vi "Coherent command pre-processing L1.vi"(9 "Data":T2, 10 "Commands & Queries":T4, 11 "Coherent laser commands L1":T3(ring)) -> (2 "Data Type":T1, 3 "Command/Query string":string, 5 "Command validated ?":bool)   [LabVIEW 2020]
uses:
  Type defs/Commands List.ctl
  Type defs/data type.ctl
  Type defs/coherent commands list.ctl
  Type defs/coherent commands.ctl
  Type defs/Command mode.ctl
  Type defs/Command syntax.ctl
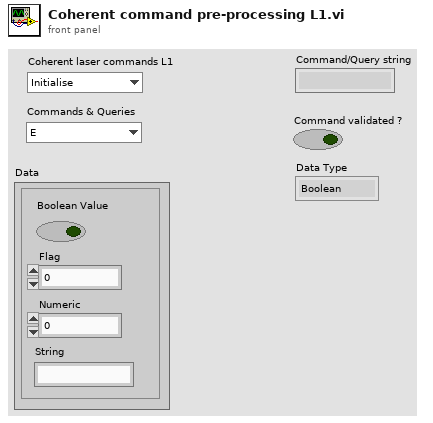
[diagram p1: front panel]
types:
  T1 = typedef "data type.ctl" = enum16{"Boolean", "Flag", "Numeric", "String", "Array"}
  T2 = cluster{"Boolean Value":bool, "Flag":i32, "Numeric":dbl, "String":string}
  T3 = enum16{"Initialise", "Get Command", "Set Command", "Close"}
  T4 = typedef "Commands List.ctl" = enum16{"E", "B", "FL", "HM", "L", "LBOH", "LBOOPT", "LFP", "PROMPT", "SM", "S", "VW", "VWS", "HB", "HBR", "REQ", "ALIGN", "K", "F", "FH", "UF", "PHLDC", "PZTMC", "PZTXC", "PZTYC", "PHLDP", "PZTMP", "PZTXP", "PZTYP", "PTRK", "MDLK", "PP", "TS", "STPRPOS", "C", "D1C", "D2C", "BT", "D1T", "D2T", "VT", "LBOT", "ET", "D1ST", "D2ST", "VST", "LBOST", "EST", "D1TD", "D2TD", "VD", "LBOD", "ED", "D1HST", "D2HST", "LRS", "D1SS", "D2SS", "VSS", "LBOSS", "ESS", "D1H", "D2H", "HH", "D1V", "D2V", "SV", "MB", "PI", "BV", "AMDLK", "PZTS", "TMAX", "TMIN", "ALIGNP", "ALIGNW", "PZTXCM", "PZTXCP", "PZTXPM", "PZTXPP", "PZTYCM", "PZTYCP", "PZTYPM", "PZTYPP", "RH", "SN", "ST", "GDDCURVE", "GDD", "GDDCURVEN", "SETCURVEN", "SETCURVEPT", "SAVECURVE", "DELCURVE", "CURVEN", "CURVEPT", "CURVE", "COMP", "HMCOMP", "GDDMAX", "GDDMIN"}
  T5 = typedef "coherent commands list.ctl" = T6[]
  T6 = typedef "coherent commands.ctl" = cluster{"Description":string, "Commands & Queries":T4, "Command Type":T7, "Data Type":T1, "Command Syntax":T8}
  T7 = typedef "Command mode.ctl" = enum16{"Read Only", "Write Only", "Read & Write"}
  T8 = typedef "Command syntax.ctl" = enum16{"Default", "Special"}
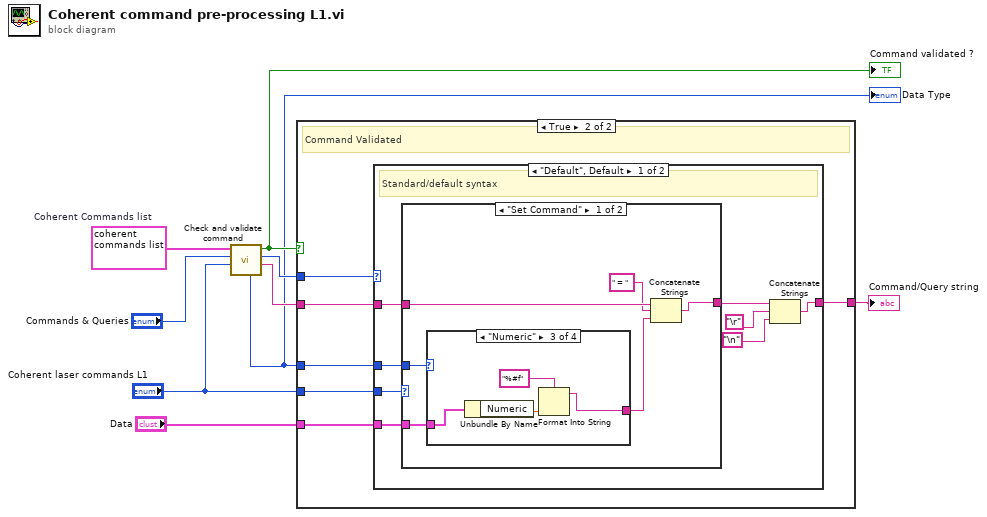
[diagram p0: block diagram]
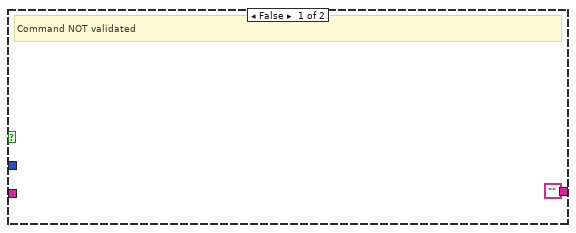
[diagram p2: hidden frame]
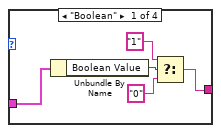
[diagram p3: hidden frame]
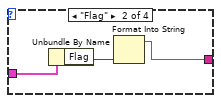
[diagram p4: hidden frame]
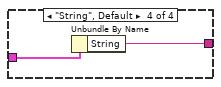
[diagram p5: hidden frame]
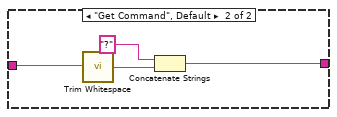
[diagram p6: hidden frame]
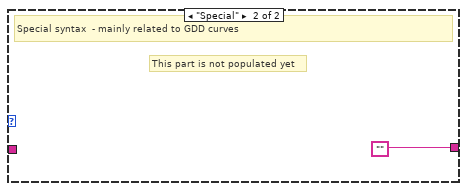
[diagram p7: hidden frame]
diagram:
  w8 = T5 [{"Description"="Changes echo settings", "Commands & Queries"=enum."E", "Command Type"=enum."Write Only", "Data Type"=enum."Boolean", "Command Syntax"=enum."Default"}, {"Description"="sets baudrate", "Commands & Queries"=enum."B", "Command Type"=enum."Write Only", "Data Type"=enum."Numeric", "Command Syntax"=enum."Default"}, {"Description"="Flash Verdi laser output below lasing threshold to allow single-frequency mode\nto recenter.\n", "Commands & Queries"=enum."FL", "Command Type"=enum."Write Only", "Data Type"=enum."Boolean", "Command Syntax"=enum."Default"}, {"Description"="Homes the tuning motor (this action can take between 3 to 30 seconds) OR provides the tuning motor status in read mode", "Commands & Queries"=enum."HM", "Command Type"=enum."Read & Write", "Data Type"=enum."Boolean", "Command Syntax"=enum."Default"}, {"Description"="changes laser mode from standby to ON or vice versa (with keyswitch in ON position). In read mode provides the Laser status\n", "Commands & Queries"=enum."L", "Command Type"=enum."Read & Write", "Data Type"=enum."Flag", "Command Syntax"=enum."Default"}, {"Description"="Turns LBO heater on/off. or indicates", "Commands & Queries"=enum."LBOH", "Command Type"=enum."Read & Write", "Data Type"=enum."Boolean", "Command Syntax"=enum."Default"}, {"Description"="Begins optimization routine.", "Commands & Queries"=enum."LBOOPT", "Command Type"=enum."Write Only", "Data Type"=enum."Boolean", "Command Syntax"=enum."Default"}, {"Description"="Turns \"CHAMELEON>\" prompt on/off.", "Commands & Queries"=enum."PROMPT", "Command Type"=enum."Write Only", "Data Type"=enum."Boolean", "Command Syntax"=enum."Default"}, {"Description"="Enables/disables search for modelocking. or displays status.", "Commands & Queries"=enum."SM", "Command Type"=enum."Read & Write", "Data Type"=enum."Boolean", "Command Syntax"=enum."Default"}, {"Description"="Changes state of the external shutter or shows the state of the shutter", "Commands & Queries"=enum."S", "Command Type"=enum."Read & Write", "Data Type"=enum."Boolean", "Command Syntax"=enum."Default"}, {"Description"="Set or display target wavelength in nanometers (nm)", "Commands & Queries"=enum."VW", "Command Type"=enum."Read & Write", "Data Type"=enum."Numeric", "Command Syntax"=enum."Default"}, {"Description"="Changes the Chameleon Ultra wavelength by the specified amount in nanometers (nm).\n", "Commands & Queries"=enum."VWS", "Command Type"=enum."Read & Write", "Data Type"=enum."Boolean", "Command Syntax"=enum."Default"}, {"Description"="When enabled, shuts the laser down if no RS-232 activity occurs within a time\nspecified by the heartbeat rate (HBR). n = 1 Enables heartbeat\n", "Commands & Queries"=enum."HB", "Command Type"=enum."Read & Write", "Data Type"=enum."Boolean", "Command Syntax"=enum."Default"}, {"Description"="Specifies to time-out period (between 1 to 100 seconds) for laser shut down in\nthe absence of RS-232 activity.", "Commands & Queries"=enum."HBR", "Command Type"=enum."Read & Write", "Data Type"=enum."Numeric", "Command Syntax"=enum."Default"}, {"Description"="Initiates recovery sequence.\nThis action can take up to 2 minutes to complete.", "Commands & Queries"=enum."REQ", "Command Type"=enum."Write Only", "Data Type"=enum."Boolean", "Command Syntax"=enum."Default"}, {"Description"="Accesses alignment mode\nn = 1 Enters alignment mode\nn = 0 Exits alignment mode", "Commands & Queries"=enum."ALIGN", "Command Type"=enum."Read & Write", "Data Type"=enum."Boolean", "Command Syntax"=enum."Default"}, {"Description"="Returns status of the keyswitch.", "Commands & Queries"=enum."K", "Command Type"=enum."Read Only", "Data Type"=enum."Boolean", "Command Syntax"=enum."Default"}, {"Description"="Returns a list of number codes of all active faults, separated by an \"&\" or\nReturns \"System OK\" if there are no active faults. Refer manual to look at the faults list\n", "Commands & Queries"=enum."F", "Command Type"=enum."Read Only", "Data Type"=enum."String", "Command Syntax"=enum."Default"}, {"Description"="Returns a list of number codes (see ?F) of all faults that have occurred since the\nlast laser on command, separated by an \"&\", or returns \"System OK\" if there are\nno latched faults. The \"laser on\" command or the EXIT button on the power\nsupply when the fault screen is active clears the fault history and fault screen.", "Commands & Queries"=enum."FH", "Command Type"=enum."Read Only", "Data Type"=enum."String", "Command Syntax"=enum."Default"}, {"Description"="Returns actual UF (Chameleon) power, nnn.nn, in milliwatts.", "Commands & Queries"=enum."UF", "Command Type"=enum."Read Only", "Data Type"=enum."Numeric", "Command Syntax"=enum."Default"}, {"Description"="Returns the status of the cavity peak hold: \n0 = Off\n1 = On\n", "Commands & Queries"=enum."PHLDC", "Command Type"=enum."Read Only", "Data Type"=enum."Boolean", "Command Syntax"=enum."Default"}, {"Description"="Returns the mode of the cavity PZT.\n0 = Auto\n1 = Manual\n", "Commands & Queries"=enum."PZTMC", "Command Type"=enum."Read Only", "Data Type"=enum."Boolean", "Command Syntax"=enum."Default"}, {"Description"="Returns the cavity PZT X (Rd) voltage, n.nn, in volts.", "Commands & Queries"=enum."PZTXC", "Command Type"=enum."Read Only", "Data Type"=enum."Numeric", "Command Syntax"=enum."Default"}, {"Description"="Returns the cavity PZT Y (Rd) voltage, n.nn, in volts.", "Commands & Queries"=enum."PZTYC", "Command Type"=enum."Read Only", "Data Type"=enum."Numeric", "Command Syntax"=enum."Default"}, {"Description"="Returns the status of the pump peak hold: \n0 = Off\n1 = On\n", "Commands & Queries"=enum."PHLDP", "Command Type"=enum."Read Only", "Data Type"=enum."Boolean", "Command Syntax"=enum."Default"}, {"Description"="Returns the mode of the pump PZT: \n0 = Auto\n1 = Manual\n", "Commands & Queries"=enum."PZTMP", "Command Type"=enum."Read Only", "Data Type"=enum."Boolean", "Command Syntax"=enum."Default"}, {"Description"="Returns pump PZT X (Rd) voltage, n.nn, in volts.", "Commands & Queries"=enum."PZTXP", "Command Type"=enum."Read Only", "Data Type"=enum."Numeric", "Command Syntax"=enum."Default"}, {"Description"="Returns pump PZT Y (Rd) voltage, n.nn, in volts.", "Commands & Queries"=enum."PZTYP", "Command Type"=enum."Read Only", "Data Type"=enum."Numeric", "Command Syntax"=enum."Default"}, {"Description"="Returns state of the PowerTrack : \n0 = Off\n1 = On", "Commands & Queries"=enum."PTRK", "Command Type"=enum."Read Only", "Data Type"=enum."Boolean", "Command Syntax"=enum."Default"}, {"Description"="Returns state of the Chameleon Ultra: \n0 = Off (Standby)\n1 = Modelocked\n2 = CW\n", "Commands & Queries"=enum."MDLK", "Command Type"=enum."Read Only", "Data Type"=enum."Flag", "Command Syntax"=enum."Default"}, {"Description"="Returns pump power setpoint as fraction of QS to CW pump band.", "Commands & Queries"=enum."PP", "Command Type"=enum."Read Only", "Data Type"=enum."Numeric", "Command Syntax"=enum."Default"}, {"Description"="Returns the tuning status:\n0 = Ready (i.e. no tuning operation being performed)\n1 = Tuning in progress\n2 = Search for Modelock in progress\n3 = Recovery operation in progress", "Commands & Queries"=enum."TS", "Command Type"=enum."Read Only", "Data Type"=enum."Flag", "Command Syntax"=enum."Default"}, {"Description"="Returns the position (counts) that the motor was last moved to for a desired\ntuning.\n", "Commands & Queries"=enum."STPRPOS", "Command Type"=enum."Read Only", "Data Type"=enum."Numeric", "Command Syntax"=enum."Default"}, {"Description"="Measured average diode current", "Commands & Queries"=enum."C", "Command Type"=enum."Read Only", "Data Type"=enum."Numeric", "Command Syntax"=enum."Default"}, {"Description"="Laser diode #1 measured current (A)", "Commands & Queries"=enum."D1C", "Command Type"=enum."Read Only", "Data Type"=enum."Numeric", "Command Syntax"=enum."Default"}, {"Description"="Laser diode #2 measured current (A)", "Commands & Queries"=enum."D2C", "Command Type"=enum."Read Only", "Data Type"=enum."Numeric", "Command Syntax"=enum."Default"}, {"Description"="Base plate temperature (deg C)", "Commands & Queries"=enum."BT", "Command Type"=enum."Read Only", "Data Type"=enum."Numeric", "Command Syntax"=enum."Default"}, {"Description"="Laser diode #1 measured temperature (deg C)", "Commands & Queries"=enum."D1T", "Command Type"=enum."Read Only", "Data Type"=enum."Numeric", "Command Syntax"=enum."Default"}, {"Description"="Laser diode #2 measured temperature (deg C)", "Commands & Queries"=enum."D2T", "Command Type"=enum."Read Only", "Data Type"=enum."Boolean", "Command Syntax"=enum."Default"}, {"Description"="Vanadate measured temperature (deg C)", "Commands & Queries"=enum."VT", "Command Type"=enum."Read Only", "Data Type"=enum."Numeric", "Command Syntax"=enum."Default"}, {"Description"="LBO temperature (deg C)", "Commands & Queries"=enum."LBOT", "Command Type"=enum."Read Only", "Data Type"=enum."Numeric", "Command Syntax"=enum."Default"}, {"Description"="Etalon measured temperature (deg C)", "Commands & Queries"=enum."ET", "Command Type"=enum."Read Only", "Data Type"=enum."Numeric", "Command Syntax"=enum."Default"}, {"Description"="Laser diode #1 set temperature (deg C)", "Commands & Queries"=enum."D1ST", "Command Type"=enum."Read Only", "Data Type"=enum."Numeric", "Command Syntax"=enum."Default"}, {"Description"="Laser diode #1 set temperature (deg C)", "Commands & Queries"=enum."D2ST", "Command Type"=enum."Read Only", "Data Type"=enum."Numeric", "Command Syntax"=enum."Default"}, {"Description"="Vanadate set temperature (deg C)", "Commands & Queries"=enum."VST", "Command Type"=enum."Read Only", "Data Type"=enum."Numeric", "Command Syntax"=enum."Default"}, {"Description"="LBO set temperature (deg C)", "Commands & Queries"=enum."LBOST", "Command Type"=enum."Read Only", "Data Type"=enum."Numeric", "Command Syntax"=enum."Default"}, {"Description"="Etalon set temperature (deg C)", "Commands & Queries"=enum."EST", "Command Type"=enum."Read Only", "Data Type"=enum."Numeric", "Command Syntax"=enum."Default"}, {"Description"="Laser diode #1 temperature servo drive setting", "Commands & Queries"=enum."D1TD", "Command Type"=enum."Read Only", "Data Type"=enum."Numeric", "Command Syntax"=enum."Default"}, {"Description"="Laser diode #2 temperature servo drive setting", "Commands & Queries"=enum."D2TD", "Command Type"=enum."Read Only", "Data Type"=enum."Numeric", "Command Syntax"=enum."Default"}, {"Description"="Vanadate temperature servo drive setting", "Commands & Queries"=enum."VD", "Command Type"=enum."Read Only", "Data Type"=enum."Numeric", "Command Syntax"=enum."Default"}, {"Description"="LBO temperature servo drive setting", "Commands & Queries"=enum."LBOD", "Command Type"=enum."Read Only", "Data Type"=enum."Numeric", "Command Syntax"=enum."Default"}, {"Description"="Etalon temperature servo drive setting", "Commands & Queries"=enum."ED", "Command Type"=enum."Read Only", "Data Type"=enum."Numeric", "Command Syntax"=enum."Default"}, {"Description"="Laser diode #1 heat sink measured temperature (deg C)", "Commands & Queries"=enum."D1HST", "Command Type"=enum."Read Only", "Data Type"=enum."Numeric", "Command Syntax"=enum."Default"}, {"Description"="Laser diode #2 heat sink measured temperature (deg C)", "Commands & Queries"=enum."D2HST", "Command Type"=enum."Read Only", "Data Type"=enum."Numeric", "Command Syntax"=enum."Default"}, {"Description"="Light loop servo status", "Commands & Queries"=enum."LRS", "Command Type"=enum."Read Only", "Data Type"=enum."Flag", "Command Syntax"=enum."Default"}, {"Description"="Diode #1 temperature servo status.", "Commands & Queries"=enum."D1SS", "Command Type"=enum."Read Only", "Data Type"=enum."Flag", "Command Syntax"=enum."Default"}, {"Description"="Diode #2 temperature servo status.", "Commands & Queries"=enum."D2SS", "Command Type"=enum."Read Only", "Data Type"=enum."Flag", "Command Syntax"=enum."Default"}, {"Description"="Vanadate temperature servo status", "Commands & Queries"=enum."VSS", "Command Type"=enum."Read Only", "Data Type"=enum."Flag", "Command Syntax"=enum."Default"}, {"Description"="LBO temperature servo status", "Commands & Queries"=enum."LBOSS", "Command Type"=enum."Read Only", "Data Type"=enum."Flag", "Command Syntax"=enum."Default"}, {"Description"="Etalon temperature servo status", "Commands & Queries"=enum."ESS", "Command Type"=enum."Read Only", "Data Type"=enum."Flag", "Command Syntax"=enum."Default"}, {"Description"="Operating hours of laser diode #1", "Commands & Queries"=enum."D1H", "Command Type"=enum."Read Only", "Data Type"=enum."Numeric", "Command Syntax"=enum."Default"}, {"Description"="Operating hours of laser diode #2", "Commands & Queries"=enum."D2H", "Command Type"=enum."Read Only", "Data Type"=enum."Numeric", "Command Syntax"=enum."Default"}, {"Description"="Power supply software", "Commands & Queries"=enum."SV", "Command Type"=enum."Read Only", "Data Type"=enum."Numeric", "Command Syntax"=enum."Default"}, {"Description"="Modem baud rate", "Commands & Queries"=enum."MB", "Command Type"=enum."Read Only", "Data Type"=enum."Numeric", "Command Syntax"=enum."Default"}, {"Description"="1 bar or 2 bar power supply", "Commands & Queries"=enum."PI", "Command Type"=enum."Read Only", "Data Type"=enum."Boolean", "Command Syntax"=enum."Default"}, {"Description"="Measured voltage across the battery.", "Commands & Queries"=enum."BV", "Command Type"=enum."Read Only", "Data Type"=enum."Numeric", "Command Syntax"=enum."Default"}, {"Description"="Auto mode lock routing", "Commands & Queries"=enum."AMDLK", "Command Type"=enum."Read Only", "Data Type"=enum."Boolean", "Command Syntax"=enum."Default"}, {"Description"="PTZ control state", "Commands & Queries"=enum."PZTS", "Command Type"=enum."Read Only", "Data Type"=enum."String", "Command Syntax"=enum."Default"}, {"Description"="Maximum available wavelength (nm)", "Commands & Queries"=enum."TMAX", "Command Type"=enum."Read Only", "Data Type"=enum."Numeric", "Command Syntax"=enum."Default"}, {"Description"="Minimum available wavelength (nm)", "Commands & Queries"=enum."TMIN", "Command Type"=enum."Read Only", "Data Type"=enum."Boolean", "Command Syntax"=enum."Default"}, {"Description"="Laser power available with alignment mode enabled (mW)", "Commands & Queries"=enum."ALIGNP", "Command Type"=enum."Read Only", "Data Type"=enum."Numeric", "Command Syntax"=enum."Default"}, {"Description"="Alignment mode laser wavelength", "Commands & Queries"=enum."ALIGNW", "Command Type"=enum."Read Only", "Data Type"=enum."Numeric", "Command Syntax"=enum."Default"}, {"Description"="Enable/disable input from front panel.", "Commands & Queries"=enum."LFP", "Command Type"=enum."Read & Write", "Data Type"=enum."Boolean", "Command Syntax"=enum."Default"}, {"Description"="X PZT position power map (% of available range)", "Commands & Queries"=enum."PZTXCM", "Command Type"=enum."Read Only", "Data Type"=enum."Numeric", "Command Syntax"=enum."Default"}, {"Description"="current cavity X PZT position (% of available range).", "Commands & Queries"=enum."PZTXCP", "Command Type"=enum."Read Only", "Data Type"=enum."Numeric", "Command Syntax"=enum."Default"}, {"Description"="X PZT position pump last power map", "Commands & Queries"=enum."PZTXPM", "Command Type"=enum."Read & Write", "Data Type"=enum."Numeric", "Command Syntax"=enum."Default"}, {"Description"="Current pump X PZT position (% of available range)", "Commands & Queries"=enum."PZTXPP", "Command Type"=enum."Read Only", "Data Type"=enum."Boolean", "Command Syntax"=enum."Default"}, {"Description"="Y PZT position power map (% of available range)", "Commands & Queries"=enum."PZTYCM", "Command Type"=enum."Read Only", "Data Type"=enum."Numeric", "Command Syntax"=enum."Default"}, {"Description"="current cavity Y PZT position (% of available range).", "Commands & Queries"=enum."PZTYCP", "Command Type"=enum."Read Only", "Data Type"=enum."Numeric", "Command Syntax"=enum."Default"}, {"Description"="Y PZT position pump last power map", "Commands & Queries"=enum."PZTYPM", "Command Type"=enum."Read Only", "Data Type"=enum."Numeric", "Command Syntax"=enum."Default"}, {"Description"="Current pump Y PZT position (% of available range)", "Commands & Queries"=enum."PZTYPP", "Command Type"=enum."Read Only", "Data Type"=enum."Boolean", "Command Syntax"=enum."Default"}, {"Description"="Relative humidity (%)", "Commands & Queries"=enum."RH", "Command Type"=enum."Read & Write", "Data Type"=enum."Numeric", "Command Syntax"=enum."Default"}, {"Description"="Chameleon serial number", "Commands & Queries"=enum."SN", "Command Type"=enum."Read Only", "Data Type"=enum."String", "Command Syntax"=enum."Default"}, {"Description"="Current status", "Commands & Queries"=enum."ST", "Command Type"=enum."Read Only", "Data Type"=enum."String", "Command Syntax"=enum."Default"}, {"Description"="GDD calibration curve number", "Commands & Queries"=enum."GDDCURVE", "Command Type"=enum."Read & Write", "Data Type"=enum."Numeric", "Command Syntax"=enum."Default"}, {"Description"="GDD value (fs2)", "Commands & Queries"=enum."GDD", "Command Type"=enum."Read & Write", "Data Type"=enum."Numeric", "Command Syntax"=enum."Default"}, {"Description"="GDD curve name", "Commands & Queries"=enum."GDDCURVEN", "Command Type"=enum."Read & Write", "Data Type"=enum."String", "Command Syntax"=enum."Default"}, {"Description"="Sets GDD curve name", "Commands & Queries"=enum."SETCURVEN", "Command Type"=enum."Read Only", "Data Type"=enum."String", "Command Syntax"=enum."Special"}, {"Description"="Curve ww point position (read manual)", "Commands & Queries"=enum."SETCURVEPT", "Command Type"=enum."Read Only", "Data Type"=enum."Numeric", "Command Syntax"=enum."Default"}, {"Description"="Save curve", "Commands & Queries"=enum."SAVECURVE", "Command Type"=enum."Write Only", "Data Type"=enum."Numeric", "Command Syntax"=enum."Default"}, {"Description"="delete curve", "Commands & Queries"=enum."DELCURVE", "Command Type"=enum."Write Only", "Data Type"=enum."Numeric", "Command Syntax"=enum."Default"}, {"Description"="Current curve name", "Commands & Queries"=enum."CURVEN", "Command Type"=enum."Read Only", "Data Type"=enum."String", "Command Syntax"=enum."Default"}, {"Description"="Curve ww point ", "Commands & Queries"=enum."CURVEPT", "Command Type"=enum."Read Only", "Data Type"=enum."Array", "Command Syntax"=enum."Special"}, {"Description"="Calibration points", "Commands & Queries"=enum."CURVE", "Command Type"=enum."Read Only", "Data Type"=enum."Array", "Command Syntax"=enum."Special"}, {"Description"="Pre compenstor enabled ?", "Commands & Queries"=enum."COMP", "Command Type"=enum."Read Only", "Data Type"=enum."Boolean", "Command Syntax"=enum."Default"}, {"Description"="Pre-compensator stepper ", "Commands & Queries"=enum."HMCOMP", "Command Type"=enum."Read Only", "Data Type"=enum."Boolean", "Command Syntax"=enum."Default"}, {"Description"="Max GDD value (at current wavelength or specified wavelength)", "Commands & Queries"=enum."GDDMAX", "Command Type"=enum."Read Only", "Data Type"=enum."Numeric", "Command Syntax"=enum."Special"}, {"Description"="Min GDD value (at current wavelength or specified wavelength)", "Commands & Queries"=enum."GDDMIN", "Command Type"=enum."Read Only", "Data Type"=enum."Numeric", "Command Syntax"=enum."Special"}]  # Coherent Commands list
  n1 = call "Check and validate command.vi"("Coherent laser commands L1"="Coherent laser commands L1", "Commands & Queries"="Commands & Queries", "Coherent Commands list"=w8) -> ("Command String"=w5:string, "Command Syntax"=w6:T8, "Command validated ?"=w7:bool, "Data Type"=w3:T1)  [unwired: 5 in]
  "Command validated ?" <- w7
  "Data Type" <- w3
  n2 = case shown="True" w7 {
    tunnel: w6 -> [_ w16]
    tunnel: w5 -> [_ w15]
    tunnel: "Coherent laser commands L1" -> [_ w14]
    tunnel: ["" w13] -> w2
    tunnel: "Data" -> [_ w12]
    tunnel: w3 -> [_ w11]
    frame False {
      # "Command NOT validated"
    }
    frame True {
      # "Command Validated"
      n3 = case shown="\"Default\", Default" w16 {
        tunnel: w15 -> [w23 _]
        tunnel: w14 -> [w24 _]
        tunnel: [w17 ""] -> w13
        tunnel: w12 -> [w22 _]
        tunnel: w11 -> [w21 _]
        frame "Default", Default {
          # "Standard/default syntax"
          n4 = case shown="\"Set Command\"" w24 {
            tunnel: w23 -> [w28 w48]
            tunnel: [w27 w45] -> w18
            tunnel: w22 -> [w29 _]
            tunnel: w21 -> [w30 _]
            frame "Set Command" {
              n5 = case shown="\"Numeric\"" w30 {
                tunnel: w29 -> [w35 w38 w41 w44]
                tunnel: [w31 w36 w39 w43] -> w25
                frame "Boolean" {
                  n6 = Unbundle By Name(w35) -> ("Boolean Value"=w34:bool)
                  n7 = Select(t="1", s=w34, f="0") -> (s? t:f=w31:string)
                }
                frame "Flag" {
                  n8 = Unbundle By Name(w38) -> ("Flag"=w37:i32)
                  n9 = Format Into String(w37) -> (resulting string=w36:string)  [unwired: 3 in, 1 out]
                }
                frame "Numeric" {
                  n10 = Unbundle By Name(w41) -> ("Numeric"=w42:dbl)
                  n11 = Format Into String(format string="%#f", w42) -> (resulting string=w39:string)  [unwired: 2 in, 1 out]
                }
                frame "String", Default {
                  n12 = Unbundle By Name(w44) -> ("String"=w43:string)
                }
              }
              n13 = Concatenate Strings(w28, " = " ("string"), w25) -> (w27:string)
            }
            frame "Get Command", Default {
              n14 = call <vilib>:"Trim Whitespace.vi"("string"=w48) -> ("trimmed string"=w46:string)  [unwired: 1 in]
              n15 = Concatenate Strings("?", w46) -> (w45:string)
            }
          }
          n16 = Concatenate Strings(w18, "\r", "\n") -> (w17:string)
        }
        frame "Special" {
          # "This part is not populated yet"
          # "Special syntax  - mainly related to GDD curves"
        }
      }
    }
  }
  "Command/Query string" <- w2
